vi "SendFFTResultsToBeckhoff.vi"(8 "error in (no error)":errorcluster, 10 "FFTResults":T1, 11 "Handle In":u32 format="%x") -> (0 "error out":errorcluster, 3 "Handle Out":u32 format="%x")   [LabVIEW 2020]
uses:
  <userlib>/Beckhoff-LabVIEW-Interface/_DependsOn/With TypeResolving/Write Sync Single TypeResolved.vi
panel:
  in  "WriteGrpSymbols 2":string[](array[string])=["192.168.0.20.1.1:851::GVL_LabviewDataShare.in_bAardvarkBoardError_labview", "192.168.0.20.1.1:851::GVL_LabviewDataShare.in_bAsic1CalibrationCompleted_labview", "192.168.0.20.1.1:851::GVL_LabviewDataShare.in_bAsic1CalibrationInProgress_labview", "192.168.0.20.1.1:851::GVL_LabviewDataShare.in_bAsic1CalibrationSuccess_labview", "192.168.0.20.1.1:851::GVL_LabviewDataShare.in_bAsic1FFTCompleted_labview", "192.168.0.20.1.1:851::GVL_LabviewDataShare.in_bAsic1FFTInProgress_labview", "192.168.0.20.1.1:851::GVL_LabviewDataShare.in_bAsic1FFTSuccess_labview", "192.168.0.20.1.1:851::GVL_LabviewDataShare.in_bAsic2CalibrationCompleted_labview", "192.168.0.20.1.1:851::GVL_LabviewDataShare.in_bAsic2CalibrationInProgress_labview", "192.168.0.20.1.1:851::GVL_LabviewDataShare.in_bAsic2CalibrationSuccess_labview", "192.168.0.20.1.1:851::GVL_LabviewDataShare.in_bAsic2FFTCompleted_labview", "192.168.0.20.1.1:851::GVL_LabviewDataShare.in_bAsic2FFTInProgress_labview", "192.168.0.20.1.1:851::GVL_LabviewDataShare.in_bAsic2FFTSuccess_labview", "192.168.0.20.1.1:851::GVL_LabviewDataShare.in_bCalResultsDBStoreSuccess_labview", "192.168.0.20.1.1:851::GVL_LabviewDataShare.in_bFFTResultsDBStoreSuccess_labview", "192.168.0.20.1.1:851::GVL_LabviewDataShare.in_bLabviewHandshakeBit", "192.168.0.20.1.1:851::GVL_LabviewDataShare.in_bLabviewResetComplete_labview", "192.168.0.20.1.1:851::GVL_LabviewDataShare.in_bLabviewResetSuccess_labview", "192.168.0.20.1.1:851::GVL_LabviewDataShare.in_bNIDaqError_labview", "192.168.0.20.1.1:851::GVL_LabviewDataShare.in_bPTC04BoardError_labview", "192.168.0.20.1.1:851::GVL_LabviewDataShare.in_bStartupInitializationCompleted_labview", "192.168.0.20.1.1:851::GVL_LabviewDataShare.in_bStartupInitializationSuccess_labview", "192.168.0.20.1.1:851::GVL_LabviewDataShare.in_strAsic1SerialNo_labview", "192.168.0.20.1.1:851::GVL_LabviewDataShare.in_strAsic2SerialNo_labview"]
  out "Write Status 8":bool
  out "Has Matched? 8":bool
  out "Write Status 7":bool
  out "Has Matched? 7":bool
  out "Write Status 6":bool
  out "Has Matched? 6":bool
  out "Write Status 5":bool
  out "Has Matched? 5":bool
  out "Write Status 4":bool
  out "Has Matched? 4":bool
  out "Write Status 2":bool
  out "Has Matched? 2":bool
  out "Write Status":bool
  out "Has Matched?":bool
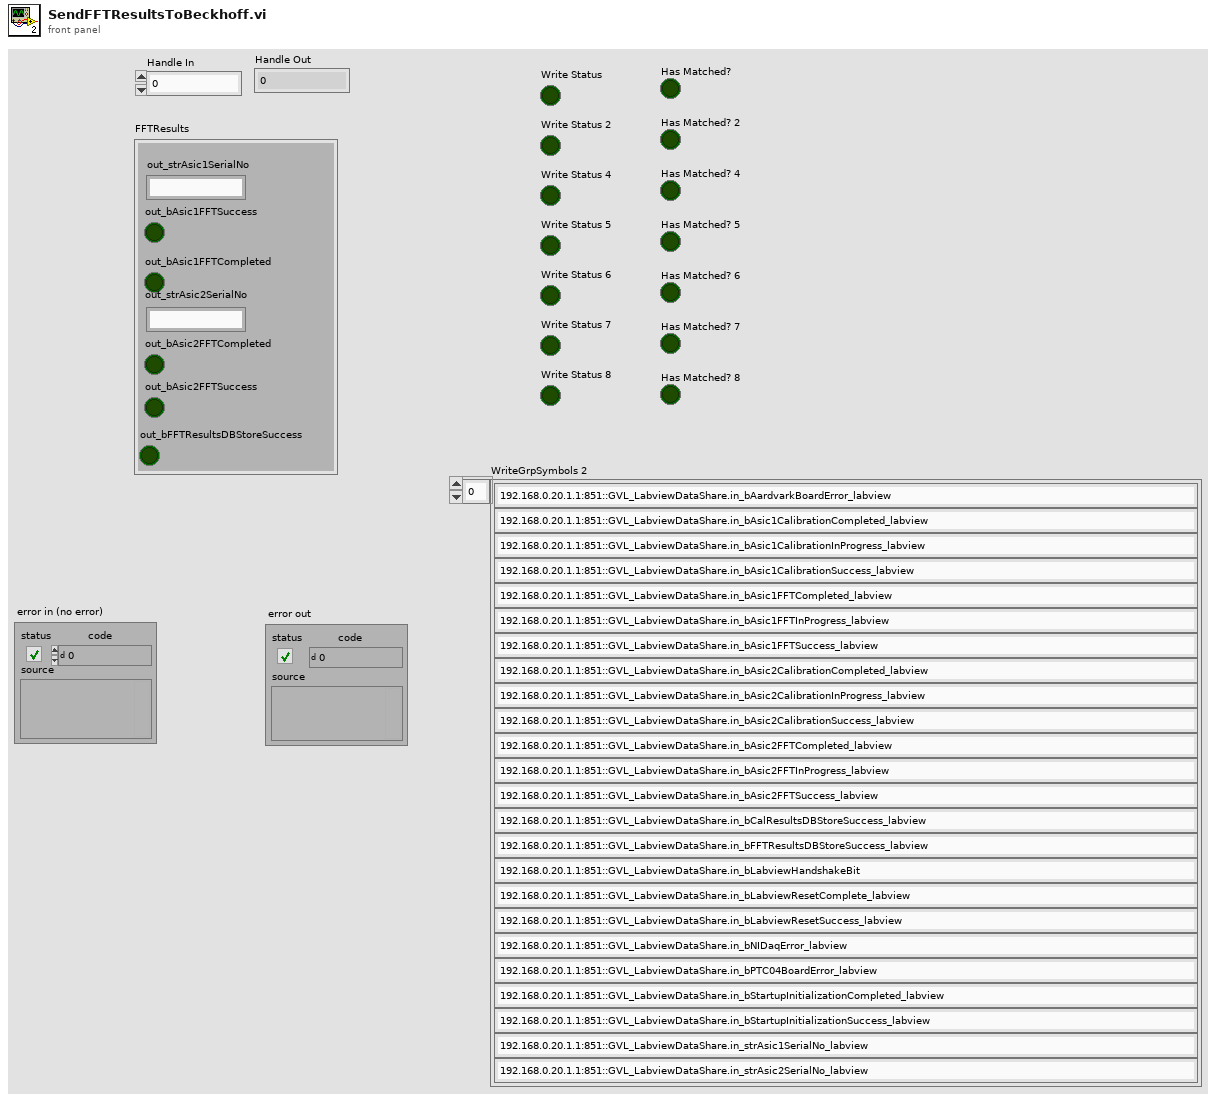
[diagram p1: front panel]
types:
  T1 = cluster{"out_strAsic1SerialNo":string, "out_bAsic1FFTSuccess":bool, "out_bAsic1FFTCompleted":bool, "out_strAsic2SerialNo":string, "out_bAsic2FFTCompleted":bool, "out_bFFTResultsDBStoreSuccess":bool, "out_bAsic2FFTSuccess":bool}
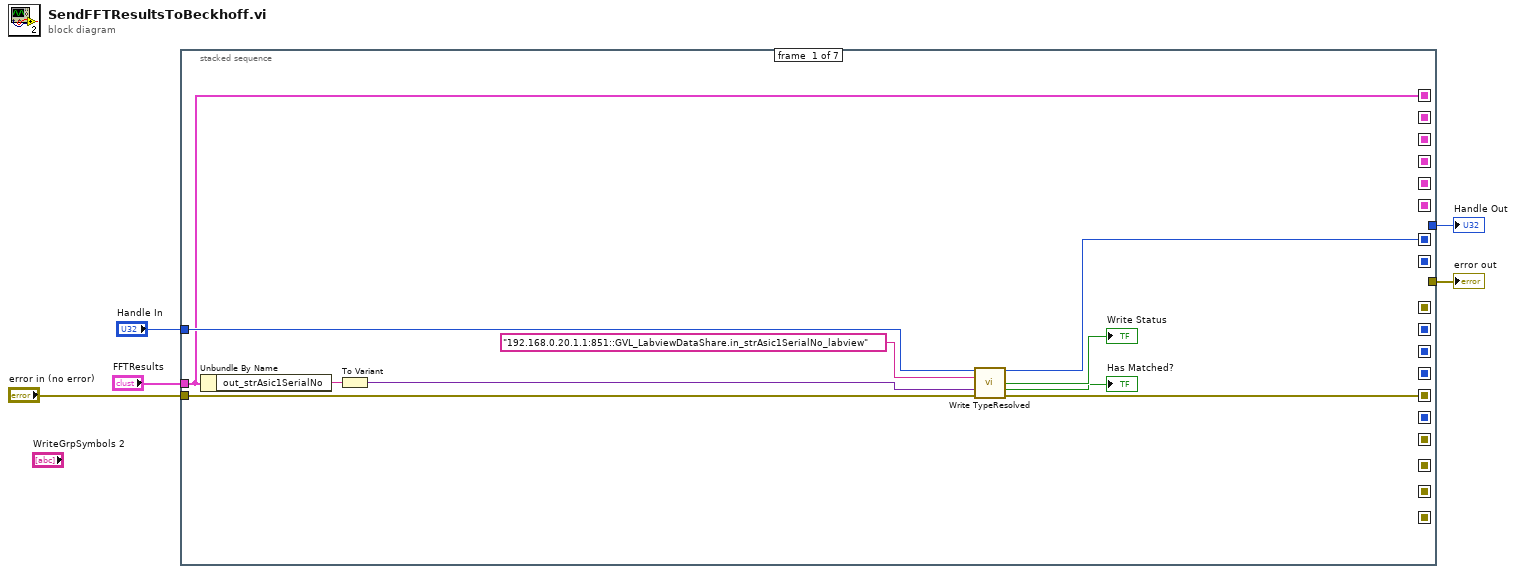
[diagram p0: block diagram]
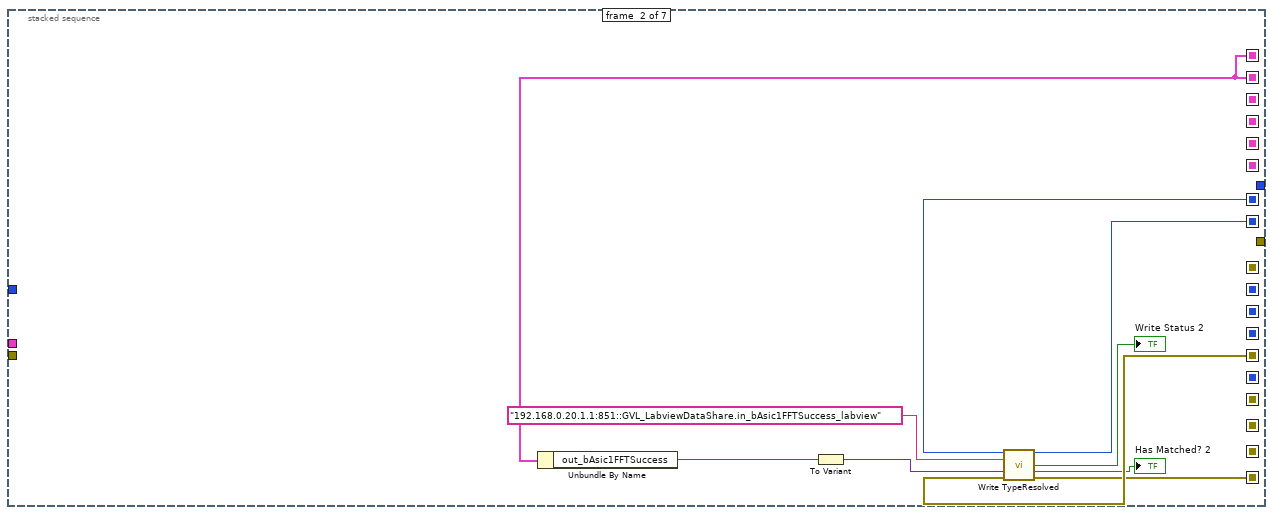
[diagram p2: hidden frame]
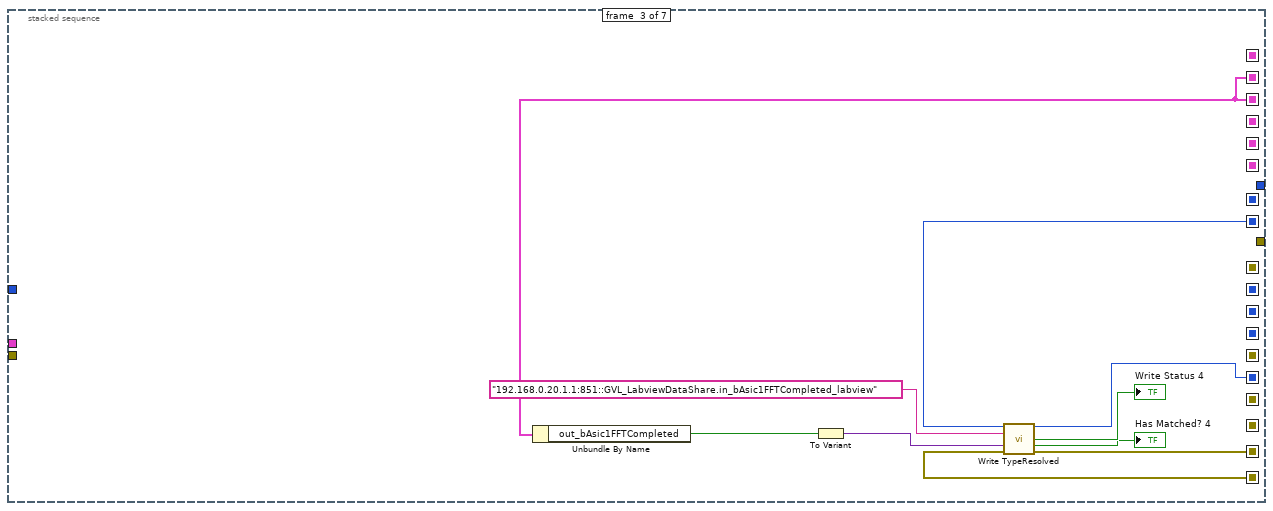
[diagram p3: hidden frame]
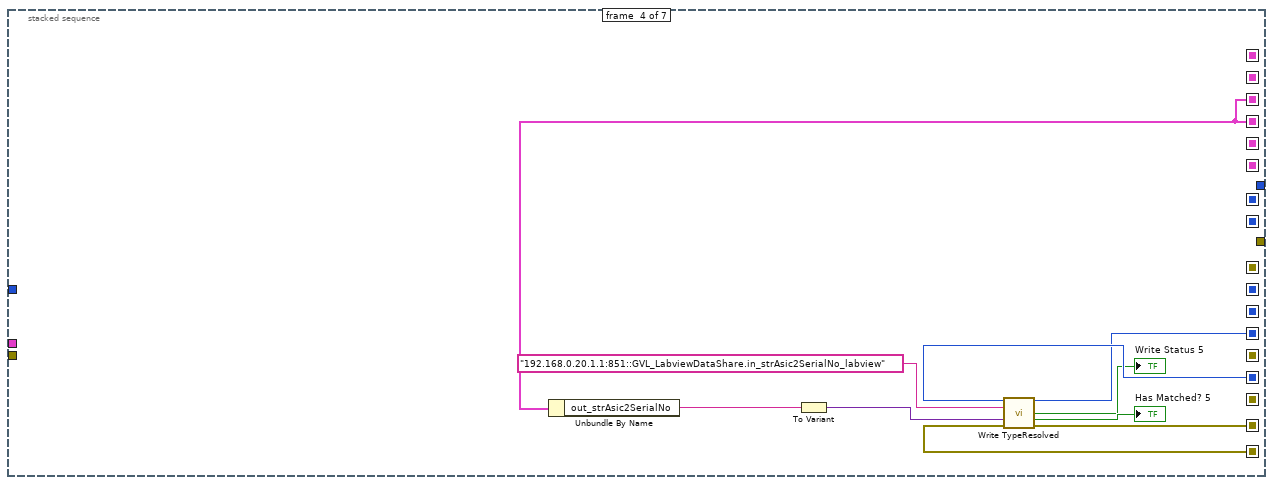
[diagram p4: hidden frame]
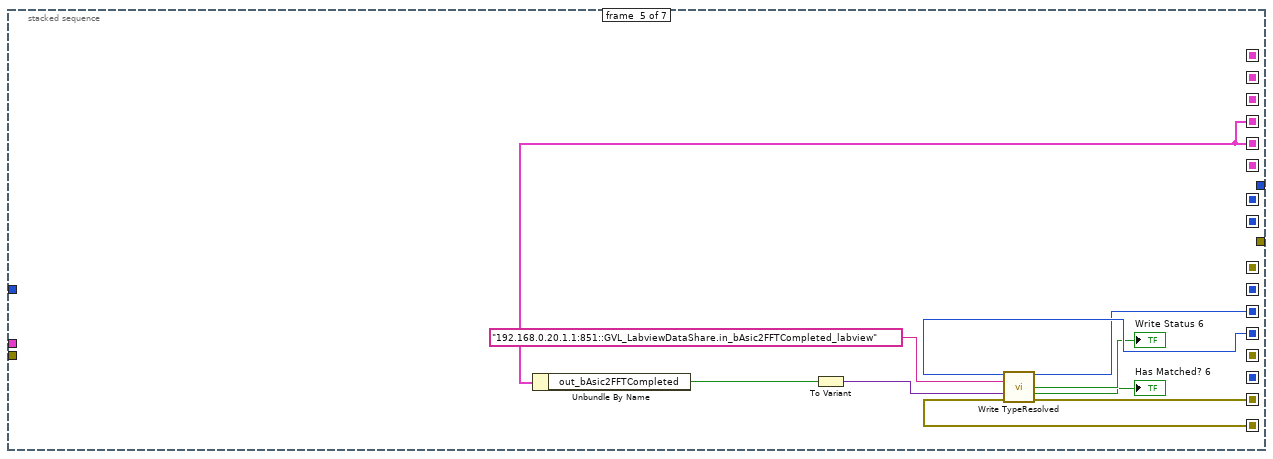
[diagram p5: hidden frame]
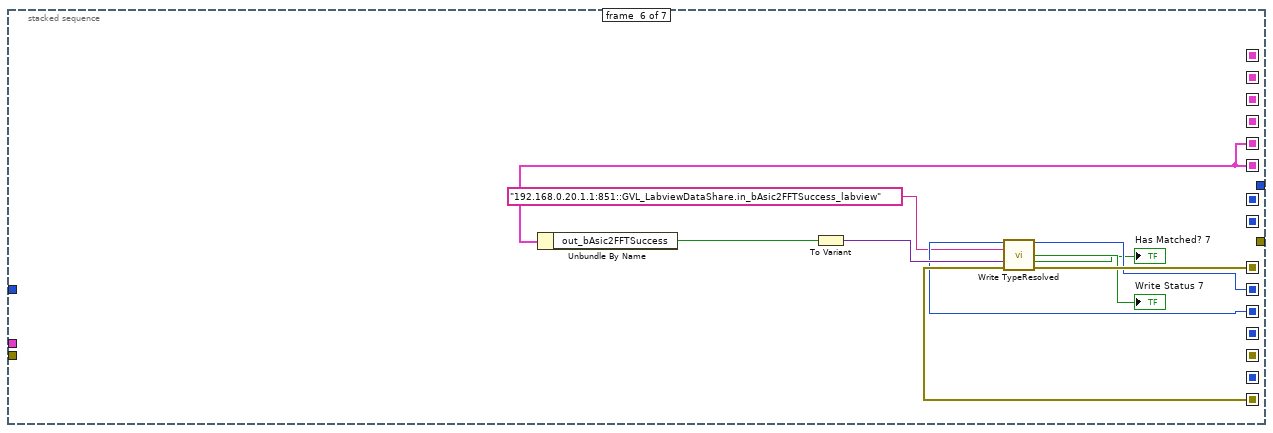
[diagram p6: hidden frame]
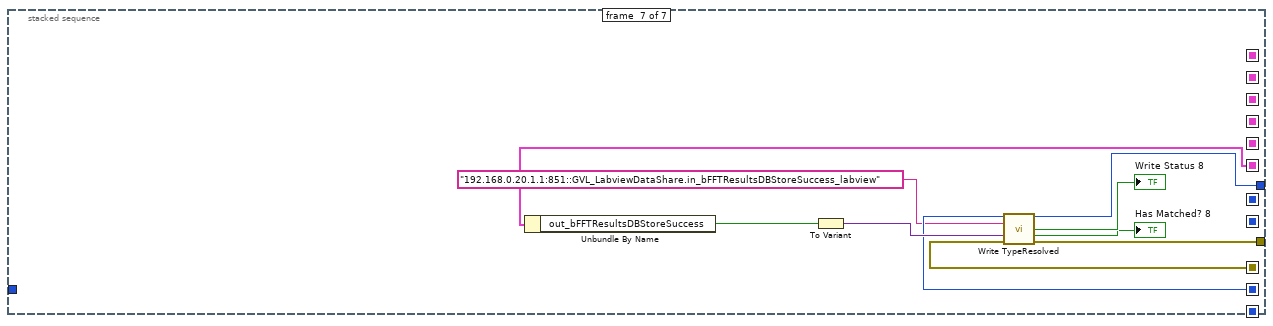
[diagram p7: hidden frame]
diagram:
  n1 = stacked-sequence {
    seq-local: [w14 _ _ _ _ _ _] -> [_ w25 _ _ _ _ _]
    seq-local: [w13 _ _ _ _ _ _] -> [_ w24 _ _ _ _ _]
    seq-local: [w9 _ _ _ _ _ _] -> [_ w19 _ _ _ _ _]
    seq-local: [_ w21 _ _ _ _ _] -> [_ _ w31 _ _ _ _]
    seq-local: [_ w20 _ _ _ _ _] -> [_ _ w30 _ _ _ _]
    seq-local: [_ w19 _ _ _ _ _] -> [_ _ w29 _ _ _ _]
    seq-local: [_ _ w32 _ _ _ _] -> [_ _ _ w41 _ _ _]
    seq-local: [_ _ w33 _ _ _ _] -> [_ _ _ w43 _ _ _]
    seq-local: [_ _ w29 _ _ _ _] -> [_ _ _ w39 _ _ _]
    seq-local: [_ _ _ w40 _ _ _] -> [_ _ _ _ w51 _ _]
    seq-local: [_ _ _ w42 _ _ _] -> [_ _ _ _ w53 _ _]
    seq-local: [_ _ _ w39 _ _ _] -> [_ _ _ _ w49 _ _]
    seq-local: [_ _ _ _ w50 _ _] -> [_ _ _ _ _ w61 _]
    seq-local: [_ _ _ _ w52 _ _] -> [_ _ _ _ _ w63 _]
    seq-local: [_ _ _ _ w49 _ _] -> [_ _ _ _ _ w59 _]
    seq-local: [_ _ _ _ _ w60 _] -> [_ _ _ _ _ _ w71]
    seq-local: [_ _ _ _ _ w62 _] -> [_ _ _ _ _ _ w73]
    seq-local: [_ _ _ _ _ w59 _] -> [_ _ _ _ _ _ w69]
    tunnel: "Handle In" -> [w15 _ _ _ _ _ _]
    tunnel: "error in (no error)" -> [w12 _ _ _ _ _ _]
    tunnel: "FFTResults" -> [w9 _ _ _ _ _ _]
    tunnel: [_ _ _ _ _ _ w70] -> w4
    tunnel: [_ _ _ _ _ _ w72] -> w3
    frame #0 {
      n2 = Unbundle By Name(w9) -> ("out_strAsic1SerialNo"=w11:string)
      n3 = To Variant(anything=w11) -> (Variant=w10:variant)
      n4 = call-poly <userlib>:"Write TypeResolved.vi"("Handle"=w15, "SymbolName"="192.168.0.20.1.1:851::GVL_LabviewDataShare.in_strAsic1SerialNo_labview", "WData"=w10, "error constant"=w12) -> ("Handle"=w14:u32, "Write Status?"=→"Write Status":bool, "Has Matched?"=→"Has Matched?":bool, "error out"=w13:errorcluster)  [unwired: 8 in]
    }
    frame #1 {
      n5 = Unbundle By Name(w19) -> ("out_bAsic1FFTSuccess"=w23:bool)
      n6 = To Variant(anything=w23) -> (Variant=w22:variant)
      n7 = call-poly <userlib>:"Write TypeResolved.vi"("Handle"=w25, "SymbolName"="192.168.0.20.1.1:851::GVL_LabviewDataShare.in_bAsic1FFTSuccess_labview", "WData"=w22, "error constant"=w24) -> ("Handle"=w21:u32, "Write Status?"=→"Write Status 2":bool, "Has Matched?"=→"Has Matched? 2":bool, "error out"=w20:errorcluster)  [unwired: 8 in]
    }
    frame #2 {
      n8 = Unbundle By Name(w29) -> ("out_bAsic1FFTCompleted"=w35:bool)
      n9 = To Variant(anything=w35) -> (Variant=w34:variant)
      n10 = call-poly <userlib>:"Write TypeResolved.vi"("Handle"=w31, "SymbolName"="192.168.0.20.1.1:851::GVL_LabviewDataShare.in_bAsic1FFTCompleted_labview", "WData"=w34, "error constant"=w30) -> ("Handle"=w32:u32, "Write Status?"=→"Write Status 4":bool, "Has Matched?"=→"Has Matched? 4":bool, "error out"=w33:errorcluster)  [unwired: 8 in]
    }
    frame #3 {
      n11 = Unbundle By Name(w39) -> ("out_strAsic2SerialNo"=w44:string)
      n12 = To Variant(anything=w44) -> (Variant=w45:variant)
      n13 = call-poly <userlib>:"Write TypeResolved.vi"("Handle"=w41, "SymbolName"="192.168.0.20.1.1:851::GVL_LabviewDataShare.in_strAsic2SerialNo_labview", "WData"=w45, "error constant"=w43) -> ("Handle"=w40:u32, "Write Status?"=→"Write Status 5":bool, "Has Matched?"=→"Has Matched? 5":bool, "error out"=w42:errorcluster)  [unwired: 8 in]
    }
    frame #4 {
      n14 = Unbundle By Name(w49) -> ("out_bAsic2FFTCompleted"=w55:bool)
      n15 = To Variant(anything=w55) -> (Variant=w54:variant)
      n16 = call-poly <userlib>:"Write TypeResolved.vi"("Handle"=w51, "SymbolName"="192.168.0.20.1.1:851::GVL_LabviewDataShare.in_bAsic2FFTCompleted_labview", "WData"=w54, "error constant"=w53) -> ("Handle"=w50:u32, "Write Status?"=→"Write Status 6":bool, "Has Matched?"=→"Has Matched? 6":bool, "error out"=w52:errorcluster)  [unwired: 8 in]
    }
    frame #5 {
      n17 = Unbundle By Name(w59) -> ("out_bAsic2FFTSuccess"=w64:bool)
      n18 = To Variant(anything=w64) -> (Variant=w65:variant)
      n19 = call-poly <userlib>:"Write TypeResolved.vi"("Handle"=w61, "SymbolName"="192.168.0.20.1.1:851::GVL_LabviewDataShare.in_bAsic2FFTSuccess_labview", "WData"=w65, "error constant"=w63) -> ("Handle"=w60:u32, "Write Status?"=→"Write Status 7":bool, "Has Matched?"=→"Has Matched? 7":bool, "error out"=w62:errorcluster)  [unwired: 8 in]
    }
    frame #6 {
      n20 = Unbundle By Name(w69) -> ("out_bFFTResultsDBStoreSuccess"=w75:bool)
      n21 = To Variant(anything=w75) -> (Variant=w74:variant)
      n22 = call-poly <userlib>:"Write TypeResolved.vi"("Handle"=w71, "SymbolName"="192.168.0.20.1.1:851::GVL_LabviewDataShare.in_bFFTResultsDBStoreSuccess_labview", "WData"=w74, "error constant"=w73) -> ("Handle"=w70:u32, "Write Status?"=→"Write Status 8":bool, "Has Matched?"=→"Has Matched? 8":bool, "error out"=w72:errorcluster)  [unwired: 8 in]
    }
  }
  "error out" <- w3
  "Handle Out" <- w4
